vi "LKIF2_DataStorageStop.vi"(8 "error in (no error)":errorcluster {"code" format="%x"}) -> (0 "error out":errorcluster {"code" format="%x"})   [LabVIEW 2013, in "Keyence LK-G5000.lvlib"]
uses:
  <instrlib>/Keyence LK-G5000/Keyence LK-G5000.lvlib
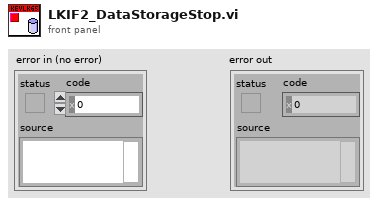
[diagram p1: front panel]
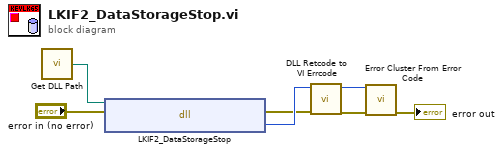
[diagram p0: block diagram]
diagram:
  n1 = call <instrlib>:"Get DLL Path.vi"() -> ("DLL Path"=w1:path)  [unwired: 1 in]
  n2 = dll-call lib="C:/Program Files/National Instruments/LabVIEW 2011/instr.lib/Keyence LK-G5000/LKIF2.dll" fn="LKIF2_DataStorageStop"(path in=w1, error in="error in (no error)") -> (error out=w2:errorcluster, "RC"=w3:i32)  [unwired: 1 in, 1 out]
  n3 = call <instrlib>:"DLL Retcode to VI Errcode.vi"("error in (no error)"=w2, "DLL Retcode"=w3) -> ("error out"=w7:errorcluster, "VI Errcode"=w6:i32)  [unwired: 8 in]
  n4 = call <vilib>:"Error Cluster From Error Code.vi"("error in (no error)"=w7, "error code (0)"=w6) -> ("error out"=→"error out":errorcluster)  [unwired: 7 in]
